vi "GUI_HPD_CCD.vi"() -> ()   [LabVIEW 2013]
uses:
  <vilib>/vision/Image Controls.llb/IMAQ Image.ctl
  Shared/GUI_Template/GUI_master/tcp new data cluster.ctl
  Shared/GUI_Template/GUI_master/tcp_new_data_event.ctl
panel:
  out "tcp data event":T1
  in  "Refresh Button":bool
  in  "Select device":string(combo)="FrogHPD"
  in  "stop":bool
  in  "trigger::1":bool caption="Trigger"
  in  "gain::1":dbl=0.001 caption="gain" min=12.0 max=400.0 format="%_4f"
  in  "centroidy::1":dbl=0.001 caption="centroid y" min=0.0 max=0.0 format="%_4f"
  in  "centroidx::1":dbl=0.001 caption="centroid x" min=0.0 max=0.0 format="%_4f"
  in  "exposure::1":dbl=0.001 caption="exposure" min=3.8e-05 max=1.0 format="%_4p"
  out "image::1":T2(plugin-control) caption="image"
  out "GUIdevice 1":string="HPD_CCD"
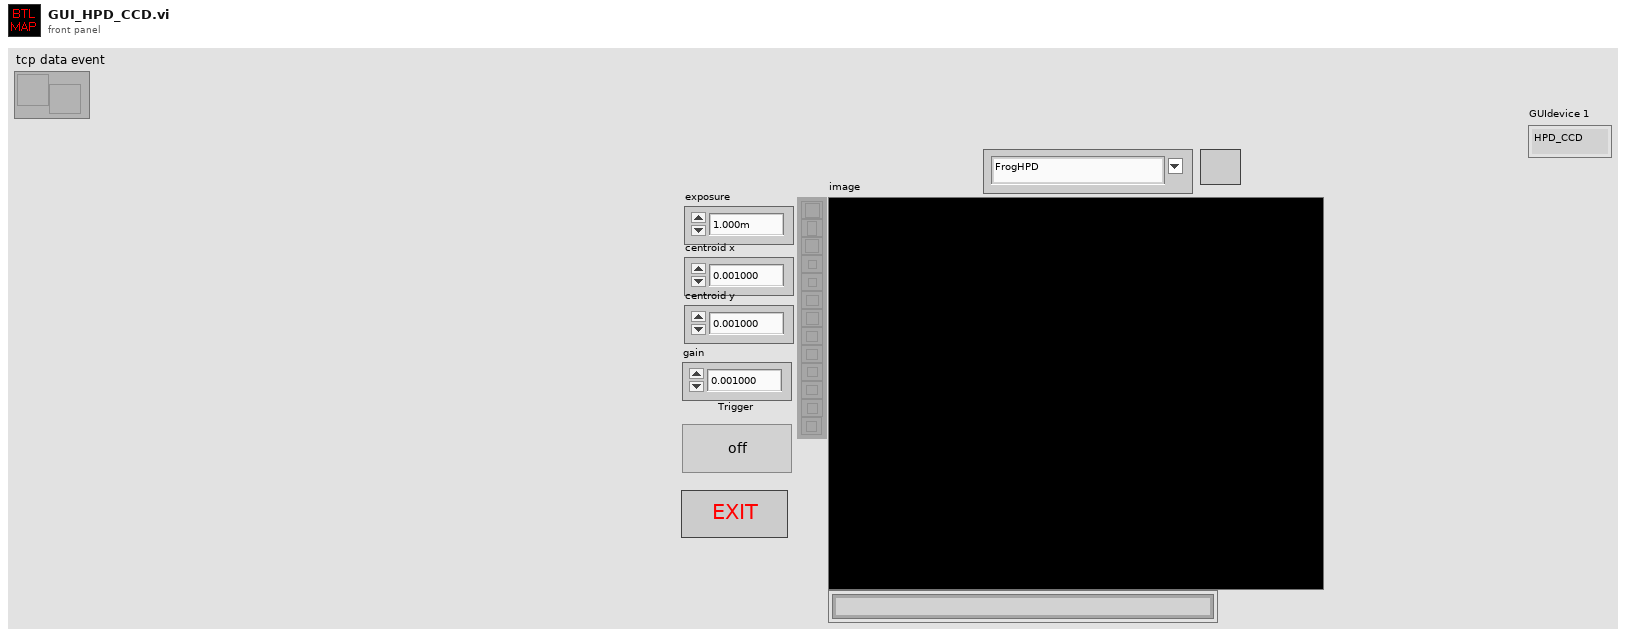
[diagram p1: front panel]
types:
  T1 = typedef "tcp_new_data_event.ctl" = refnum<user-event>
  T2 = typedef "IMAQ Image.ctl" = refnum<image>
  T3 = enum32{"invalid app kind", "Development System", "Run Time System", "Student Edition", "Embedded LabVIEW", "Evaluation", "Custom"}
  T4 = typedef "tcp new data cluster.ctl" = cluster{"EventEnum":enum16{"new data", "connection status update"}, "Device name":string}
  T5 = enum32{"Invalid", "Standard", "Closed", "Hidden", "Minimized", "Maximized"}
  T6 = cluster{"Core":cluster{"Current VI Reference":refnum<vi>, "Close Panel on Exit?":bool}, "Your Boolean data":bool, "Your string data":string, "SuperGUI":cluster{"STOP queue":refnum<queue>, "SuperGUI ref":refnum<vi>}}
  T7 = cluster{"STOP queue":refnum<queue>, "SuperGUI ref":refnum<vi>}
  T8 = cluster{"Current VI Reference":refnum<vi>, "Close Panel on Exit?":bool}
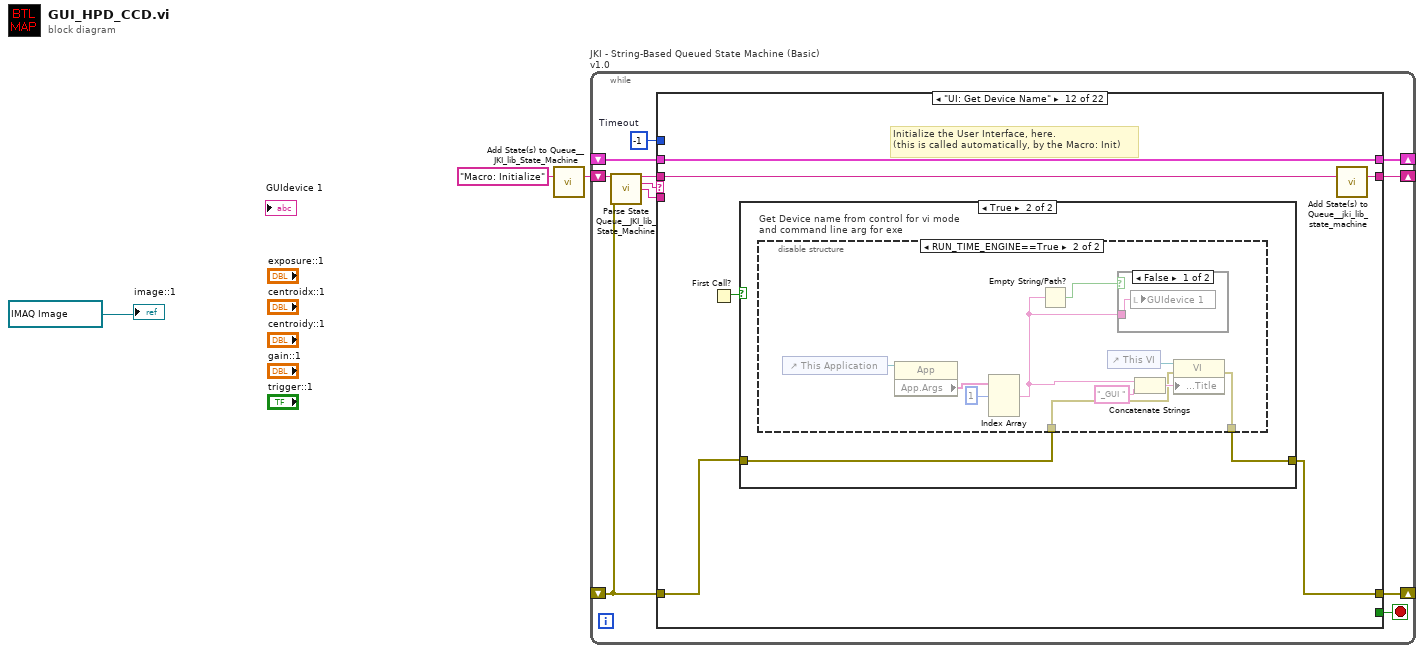
[diagram p0: block diagram]
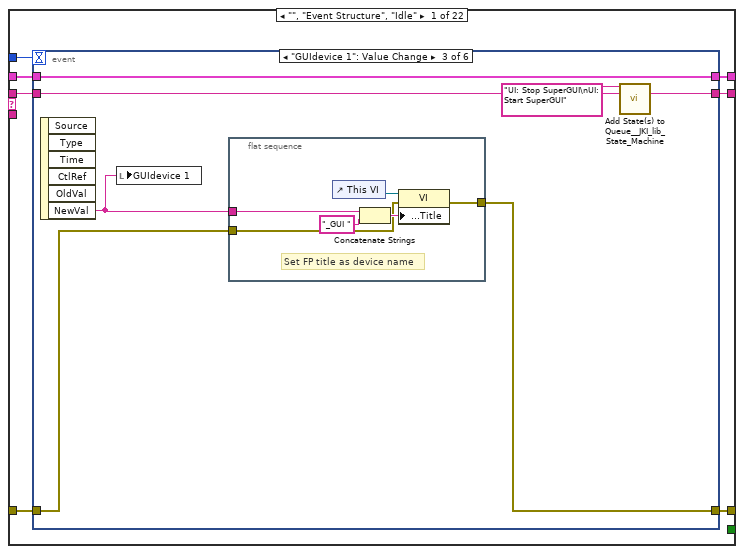
[diagram p2: hidden frame]
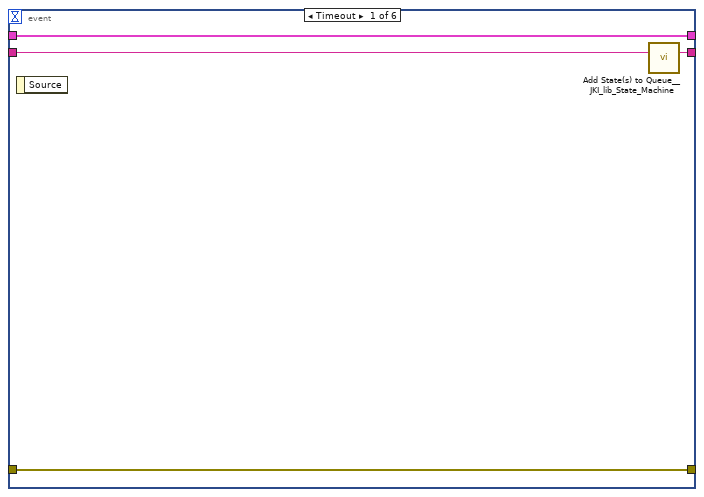
[diagram p3: hidden frame]
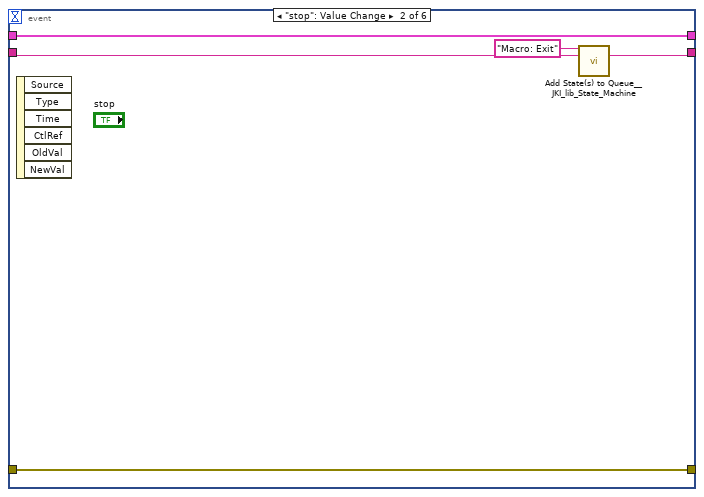
[diagram p4: hidden frame]
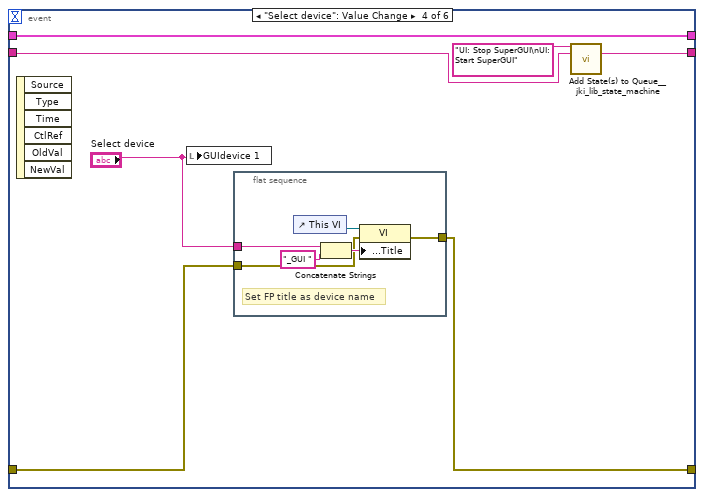
[diagram p5: hidden frame]
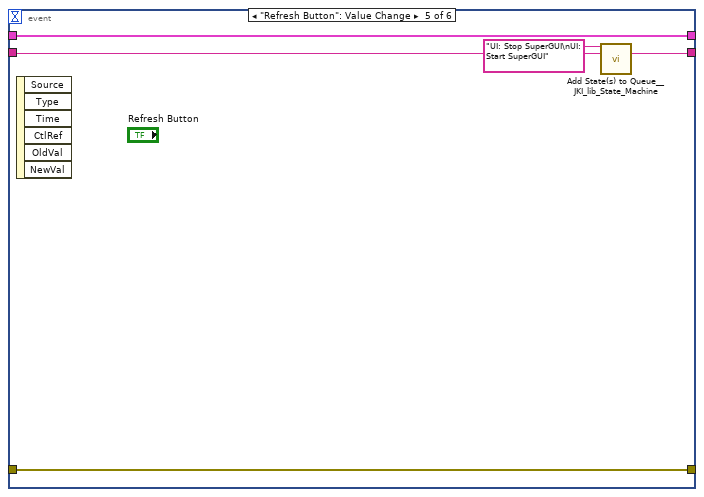
[diagram p6: hidden frame]
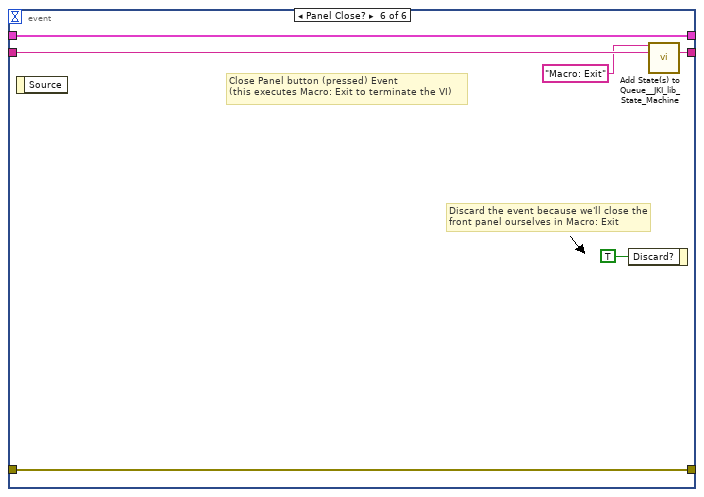
[diagram p7: hidden frame]
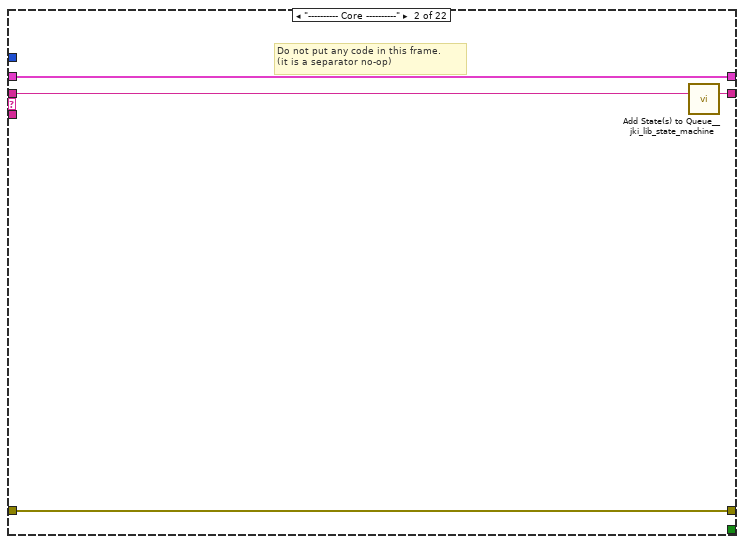
[diagram p8: hidden frame]
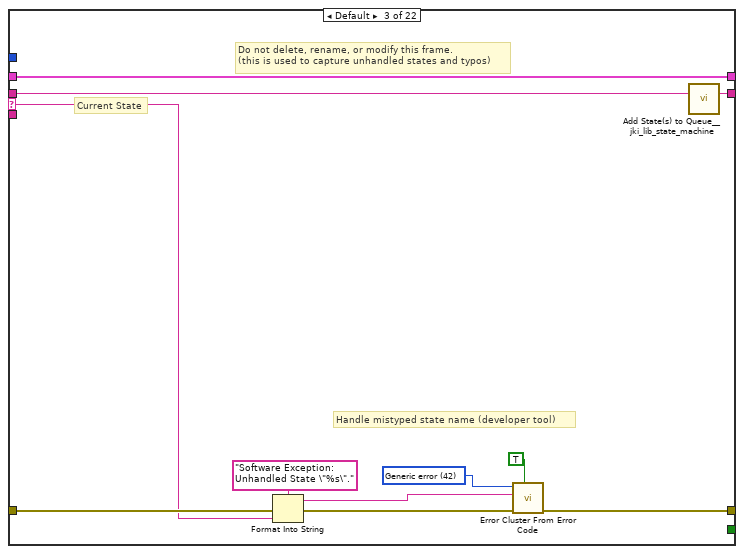
[diagram p9: hidden frame]
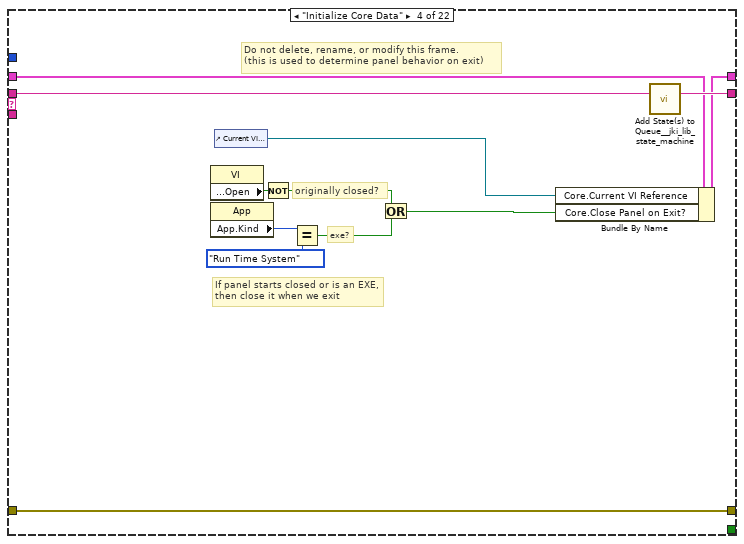
[diagram p10: hidden frame]
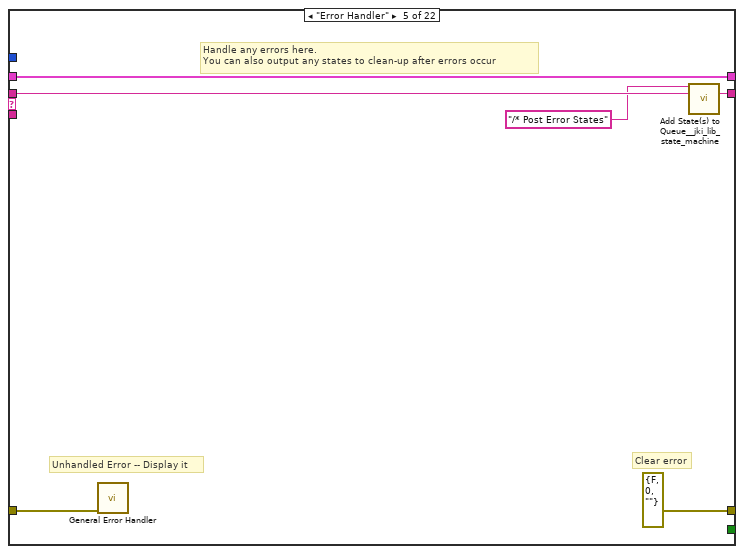
[diagram p11: hidden frame]
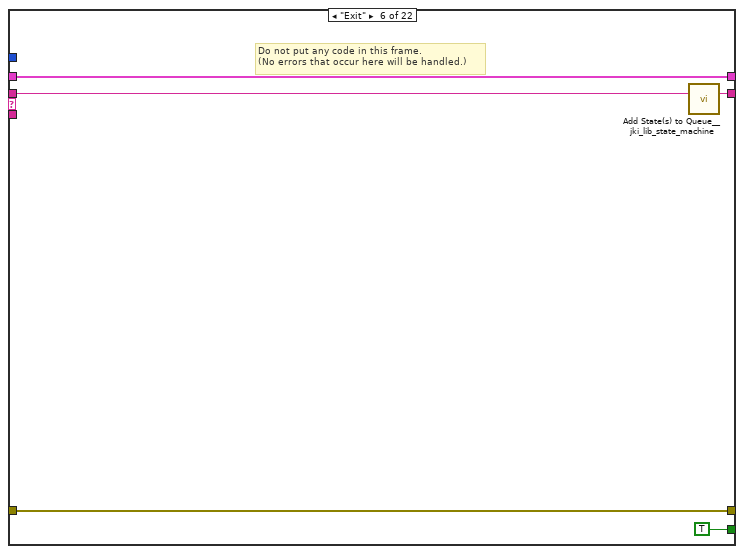
[diagram p12: hidden frame]
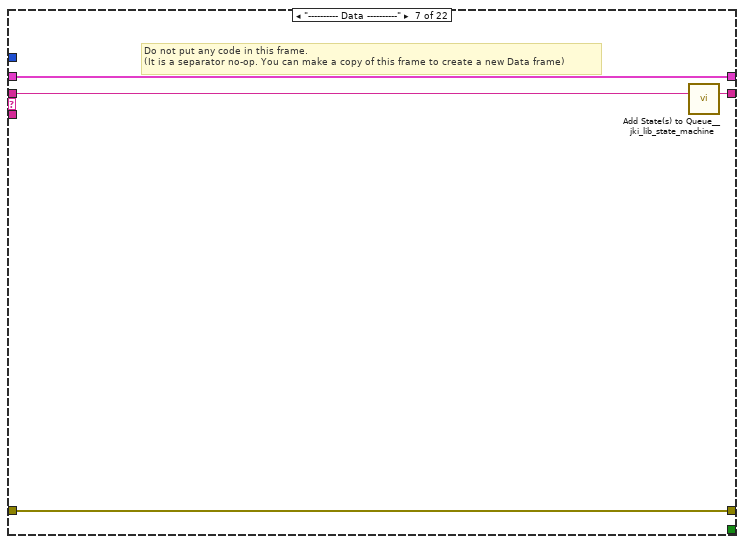
[diagram p13: hidden frame]
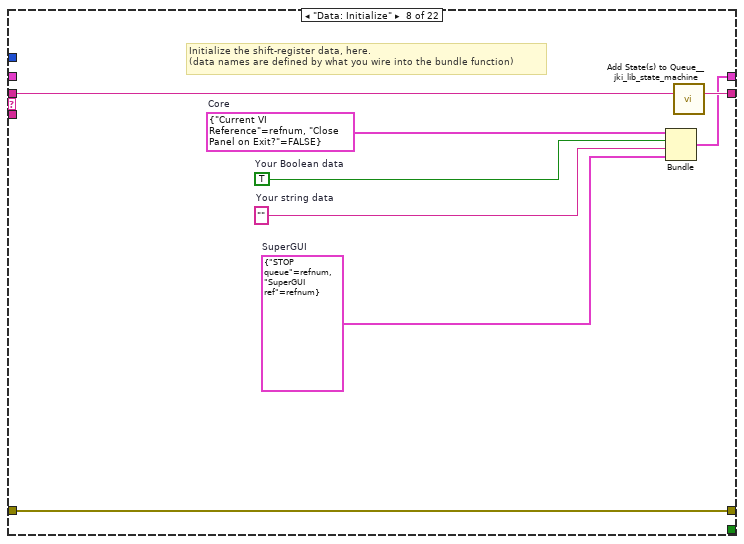
[diagram p14: hidden frame]
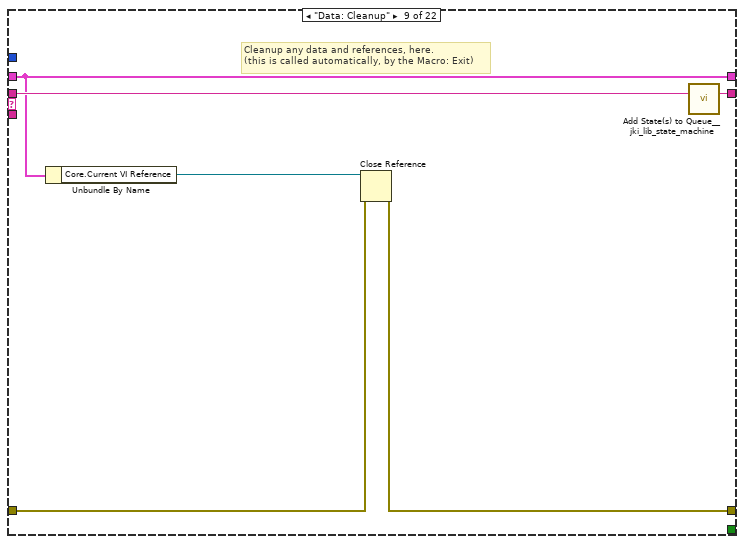
[diagram p15: hidden frame]
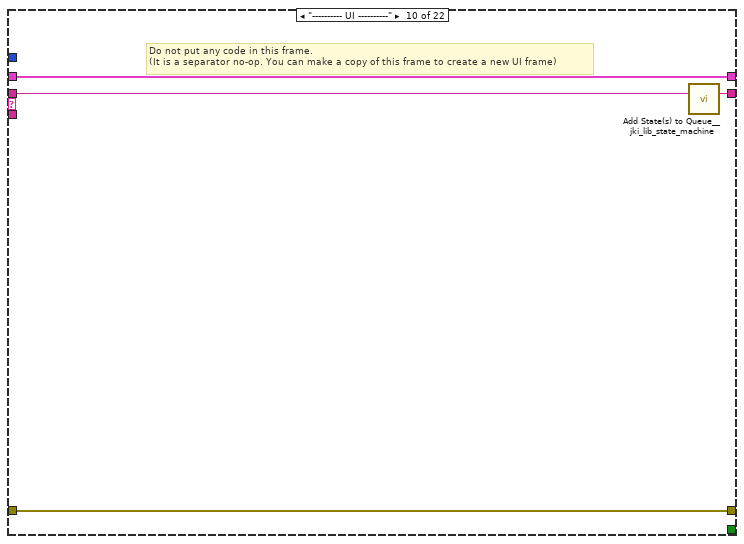
[diagram p16: hidden frame]
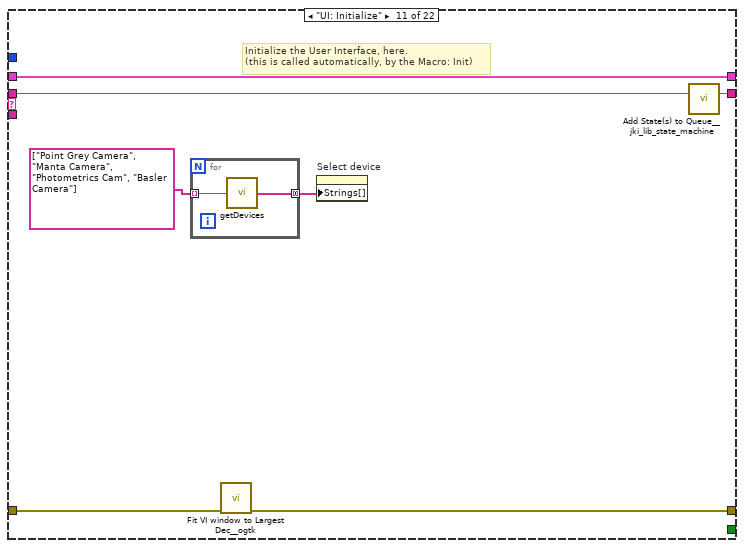
[diagram p17: hidden frame]
diagram:
  n1 = call <vilib>:"Add State(s) to Queue__JKI_lib_State_Machine.vi"("State(s) in (\"\")"="Macro: Initialize") -> ("States Out"=w2:string)  [unwired: 14 in]
  n2 = while "JKI - String-Based Queued State Machine (Basic) v1.0" {
    shift-right: [w7] -> _
    shift-left: _ -> [w6]
    shift-right: [w10] -> _
    shift-left: _ -> [w4]
    shift-right: [w9] -> _
    shift-left: w2 -> [w11]
    stop <- w8 stop-if-true
    w5 = -1  # Timeout
    n3 = call <vilib>:"Parse State Queue__JKI_lib_State_Machine.vi"("State Queue"=w11, "Error In (no error)"=w4) -> ("Remaining States"=w13:string, "Current State"=w14:string, "Arguments"=w12:string)  [unwired: 11 in]
    n4 = case shown="\"UI: Get Device Name\"" w14 {
      selector: w14 -> [_ _ w72 _ _ _ _ _ _ _ _ _ _ _ _ _ _ _ _ _ _ _]
      tunnel: w13 -> [w21 w71 w76 w94 w100 w105 w109 w117 w123 w127 w134 w142 w177 w185 w191 w202 w228 w233 w243 w247 w251 w255]
      tunnel: w12 -> [_ _ _ _ _ _ _ _ _ _ _ _ _ _ w186 w196 _ _ _ _ _ _]
      tunnel: w6 -> [w19 w68 w74 w85 w97 w103 w106 _ w118 w124 w132 w140 w168 w180 w189 w198 w225 w230 w240 w244 w248 w252]
      tunnel: [w18 w69 w78 w91 errorcluster {"status"=FALSE, "code"=0, "source"=""} ("error out") w102 w107 w114 w119 w125 w130 w137 w161 w178 w187 w199 w226 w231 w241 w245 w249 w253] -> w10
      tunnel: w4 -> [w17 w69 w77 w91 w96 w102 w107 w114 w120 w125 w131 w138 w162 w179 w188 w200 w226 w231 w241 w245 w249 w253]
      tunnel: [w20 w70 w75 w93 w99 w104 w108 w116 w122 w126 w133 w141 w176 w184 w190 w201 w227 w232 w242 w246 w250 w254] -> w9
      tunnel: [_ _ _ _ _ TRUE _ _ _ _ _ _ _ _ _ _ _ _ _ _ _ _] -> w8
      tunnel: [w16 w68 w74 w92 w97 w103 w106 w115 w118 w124 w132 w140 w167 w180 w189 w198 w225 w230 w240 w244 w248 w252] -> w7
      tunnel: w5 -> [w15 _ _ _ _ _ _ _ _ _ _ _ _ _ _ _ _ _ _ _ _ _]
      frame "", "Event Structure", "Idle" {
        n5 = event shown="[2] \"GUIdevice 1\": Value Change" {
          selector: _ -> [_ _ _ _ _ _]
          dyn-events: _ -> [_ _ _ _ _ _]
          timeout: w15 -> [_ _ _ _ _ _]
          tunnel: w21 -> [w25 w28 w34 w46 w59 w67]
          tunnel: [w24 w27 w33 w45 w58 w66] -> w20
          tunnel: w19 -> [w22 w30 w37 w50 w61 w64]
          tunnel: [w23 w29 w35 w48 w60 w65] -> w18
          tunnel: w17 -> [w23 w29 w36 w49 w60 w65]
          tunnel: [w22 w30 w37 w50 w61 w64] -> w16
          event Timeout {
            n6 = event-data() -> ()  [unwired: 1 in, 1 out]
            n7 = call <vilib>:"Add State(s) to Queue__JKI_lib_State_Machine.vi"("State(s) in (\"\")"=w25) -> ("States Out"=w24:string)  [unwired: 14 in]
          }
          event "stop": Value Change {
            n8 = event-data() -> ()  [unwired: 1 in, 6 out]
            n9 = call <vilib>:"Add State(s) to Queue__JKI_lib_State_Machine.vi"("State(s) in Front (\"\")"="Macro: Exit", "State(s) in (\"\")"=w28) -> ("States Out"=w27:string)  [unwired: 13 in]
          }
          event "GUIdevice 1": Value Change {
            n10 = event-data() -> ("NewVal"=w31:string)  [unwired: 1 in, 5 out]
            n11 = local write "GUIdevice 1"(w31) -> ()
            n12 = flat-sequence {
              tunnel: [w40] -> w35
              tunnel: w36 -> [w39]
              tunnel: w31 -> [w38]
              frame #0 {
                # "Set FP title as device name"
                n13 = control-ref of="This VI"() -> (w43:refnum<vi>)
                n14 = Concatenate Strings(w38, "_GUI ") -> (w42:string)
                n15 = property class="VI"(reference=w43, error in=w39, "Front Panel.Title"=w42) -> (error out=w40:errorcluster)  [unwired: 1 out]
              }
            }
            n16 = call <vilib>:"Add State(s) to Queue__JKI_lib_State_Machine.vi"("State(s) in Front (\"\")"="UI: Stop SuperGUI\nUI: Start SuperGUI", "State(s) in (\"\")"=w34) -> ("States Out"=w33:string)  [unwired: 13 in]
          }
          event "Select device": Value Change {
            n17 = event-data() -> ()  [unwired: 1 in, 6 out]
            n18 = local write "GUIdevice 1"("Select device") -> ()
            n19 = flat-sequence {
              tunnel: [w53] -> w48
              tunnel: w49 -> [w52]
              tunnel: "Select device" -> [w51]
              frame #0 {
                # "Set FP title as device name"
                n20 = control-ref of="This VI"() -> (w56:refnum<vi>)
                n21 = Concatenate Strings(w51, "_GUI ") -> (w55:string)
                n22 = property class="VI"(reference=w56, error in=w52, "Front Panel.Title"=w55) -> (error out=w53:errorcluster)  [unwired: 1 out]
              }
            }
            n23 = call <vilib>:"Add State(s) to Queue__jki_lib_state_machine.vi"("State(s) in Front (\"\")"="UI: Stop SuperGUI\nUI: Start SuperGUI", "State(s) in (\"\")"=w46) -> ("States Out"=w45:string)  [unwired: 13 in]
          }
          event "Refresh Button": Value Change {
            n24 = event-data() -> ()  [unwired: 1 in, 6 out]
            n25 = call <vilib>:"Add State(s) to Queue__JKI_lib_State_Machine.vi"("State(s) in Front (\"\")"="UI: Stop SuperGUI\nUI: Start SuperGUI", "State(s) in (\"\")"=w59) -> ("States Out"=w58:string)  [unwired: 13 in]
          }
          event Panel Close? {
            # "Discard the event because we'll close the front panel ourselves in Macro: Exit"
            # "Close Panel button (pressed) Event\n(this executes Macro: Exit to terminate the VI)"
            n26 = event-data() -> ()  [unwired: 1 in, 1 out]
            n27 = event-data("Discard?"=TRUE) -> ()  [unwired: 1 in, 1 out]
            n28 = call <vilib>:"Add State(s) to Queue__JKI_lib_State_Machine.vi"("State(s) in Front (\"\")"="Macro: Exit", "State(s) in (\"\")"=w67) -> ("States Out"=w66:string)  [unwired: 13 in]
          }
        }
      }
      frame "---------- Core ----------" {
        # "Do not put any code in this frame.\n(it is a separator no-op)"
        n29 = call <vilib>:"Add State(s) to Queue__jki_lib_state_machine.vi"("State(s) in (\"\")"=w71) -> ("States Out"=w70:string)  [unwired: 14 in]
      }
      frame Default {
        w81 = 42 items=["No error", "Argument error", "Memory is full", "Out of zone", "End of file", "File already open", "Generic file I/O error", "File not found", "File permission error", "Disk is full", "Duplicate path", "Too many files open", "System feature not enabled", "Resource file not found", "Cannot add resource", "Resource not found", "Image not found", "Image memory error", "Pen does not exist", "Config type invalid", "Config token not found", "Config parse error", "Config memory error", "Bad external code format", "Bad external code offset", "External code not present", "Null window", "Destroy window error", "Null menu", "Print aborted", "Bad print record", "Print driver error", "Windows error during printing", "Memory error during printing", "Print dialog error", "Generic print error", "Invalid device refnum", "Device not found", "Device parameter error", "Device unit error", "Cannot open device", "Device call aborted", "Generic error", "Cancelled by user", "Object ID too low", "Object ID too high", "Object not in heap", "Unknown heap", "Unknown object (invalid DefProc)", "Unknown object (DefProc not in table)", "Message out of range", "Invalid (null) method", "Unknown message", "Manager call not supported", "Bad address", "Network operation in progress", "Network operation timed out", "Connection is busy", "Network attribute not supported", "Network error", "Address in use", "System out of memory", "Connection aborted", "Connection refused", "Not connected", "Already connected", "Connection closed", "Initialization error (interapplication manager)", "Bad occurrence", "Wait on unbound occurrence handler", "Occurrence queue overflow", "Datalog type conflict", "Unused", "Unrecognized type (interapplication manager)", "Memory corrupt", "Failed to make temporary DLL", "Old CIN version", "Drag socket not found", "Failed to load drop-object", "Failed to register OLE object", "Failed to release OLE object", "Format specifier type mismatch", "Unknown format specifier", "Too few format specifiers", "Too many format specifiers", "Scan failed", "Newer CIN version", "Error converting to variant", "Runtime menu error", "Password tampered", "Variant attribute not found", "Incompatible variant data type", "Event data is not available", "Event Store is not present", "Occurrence is not found", "Event Queue is not created", "Event info is not available", "Refnum passed is NULL", "Error retrieving Class GUID", "Error retrieving CoClass GUID", "Error retrieving TypeLib GUID.", "Bad built application magic bytes.", "Specific driver is different from the specific driver associated with the Logical Name.", "There is no session opened to the class driver.", "Max Error", "MAX - Error with config objects", "MAX - Error loading configuration", "MAX - Group not supported"]
        # "Current State"
        # "Do not delete, rename, or modify this frame.\n(this is used to capture unhandled states and typos)"
        # "Handle mistyped state name (developer tool)"
        n30 = Format Into String(format string="Software Exception: Unhandled State \"%s\"." ("message"), error in=w77, w72) -> (resulting string=w80:string, error out=w79:errorcluster)  [unwired: 1 in]
        n31 = call <vilib>:"Error Cluster From Error Code.vi"("show call chain? (False)"=TRUE, "error in (no error)"=w79, "error message (\"\")"=w80, "error code (0)"=w81) -> ("error out"=w78:errorcluster)  [unwired: 5 in]
        n32 = call <vilib>:"Add State(s) to Queue__jki_lib_state_machine.vi"("State(s) in (\"\")"=w76) -> ("States Out"=w75:string)  [unwired: 14 in]
      }
      frame "Initialize Core Data" {
        # "Do not delete, rename, or modify this frame.\n(this is used to determine panel behavior on exit)"
        # "originally closed?"
        # "exe?"
        # "If panel starts closed or is an EXE, then close it when we exit"
        n33 = property class="VI"() -> ("Front Panel.Open"=w90:bool)  [unwired: 2 in, 2 out]
        n34 = property class="App"() -> ("App.Kind"=w89:T3)  [unwired: 2 in, 2 out]
        n35 = control-ref of="Current VI Reference"() -> (w83:refnum<vi>)
        n36 = Not(x=w90) -> (.not. x?=w87:bool)
        n37 = Equal?(x=w89, y=T3."Run Time System" ("Application:Kind")) -> (x = y?=w86:bool)
        n38 = Or(x=w87, y=w86) -> (x .or. y?=w84:bool)
        n39 = Bundle By Name(cluster=w85, "Core.Current VI Reference"=w83, "Core.Close Panel on Exit?"=w84) -> (w92:T6)
        n40 = call <vilib>:"Add State(s) to Queue__jki_lib_state_machine.vi"("State(s) in (\"\")"=w94) -> ("States Out"=w93:string)  [unwired: 14 in]
      }
      frame "Error Handler" {
        # "Unhandled Error -- Display it"
        # "Handle any errors here.\nYou can also output any states to clean-up after errors occur"
        # "Clear error"
        n41 = call <vilib>:"General Error Handler.vi"("error in (no error)"=w96) -> ()  [unwired: 10 in, 5 out]
        n42 = call <vilib>:"Add State(s) to Queue__jki_lib_state_machine.vi"("State(s) in Front (\"\")"="/* Post Error States", "State(s) in (\"\")"=w100) -> ("States Out"=w99:string)  [unwired: 13 in]
      }
      frame "Exit" {
        # "Do not put any code in this frame.\n(No errors that occur here will be handled.)"
        n43 = call <vilib>:"Add State(s) to Queue__jki_lib_state_machine.vi"("State(s) in (\"\")"=w105) -> ("States Out"=w104:string)  [unwired: 14 in]
      }
      frame "---------- Data ----------" {
        # "Do not put any code in this frame.\n(It is a separator no-op. You can make a copy of this frame to create a new Data frame)"
        n44 = call <vilib>:"Add State(s) to Queue__jki_lib_state_machine.vi"("State(s) in (\"\")"=w109) -> ("States Out"=w108:string)  [unwired: 14 in]
      }
      frame "Data: Initialize" {
        w110 = T7 {"STOP queue"=refnum, "SuperGUI ref"=refnum}  # SuperGUI
        w111 = T8 {"Current VI Reference"=refnum, "Close Panel on Exit?"=FALSE}  # Core
        w113 = TRUE  # Your Boolean data
        w112 = ""  # Your string data
        # "Initialize the shift-register data, here.\n(data names are defined by what you wire into the bundle function)"
        n45 = Bundle("Core"=w111, "Your Boolean data"=w113, "Your string data"=w112, "SuperGUI"=w110) -> (w115:T6)  [unwired: 1 in]
        n46 = call <vilib>:"Add State(s) to Queue__jki_lib_state_machine.vi"("State(s) in (\"\")"=w117) -> ("States Out"=w116:string)  [unwired: 14 in]
      }
      frame "Data: Cleanup" {
        # "Cleanup any data and references, here.\n(this is called automatically, by the Macro: Exit)"
        n47 = Unbundle By Name(w118) -> ("Core.Current VI Reference"=w121:refnum<vi>)
        n48 = Close Reference(reference=w121, error in (no error)=w120) -> (error out=w119:errorcluster)
        n49 = call <vilib>:"Add State(s) to Queue__jki_lib_state_machine.vi"("State(s) in (\"\")"=w123) -> ("States Out"=w122:string)  [unwired: 14 in]
      }
      frame "---------- UI ----------" {
        # "Do not put any code in this frame.\n(It is a separator no-op. You can make a copy of this frame to create a new UI frame)"
        n50 = call <vilib>:"Add State(s) to Queue__jki_lib_state_machine.vi"("State(s) in (\"\")"=w127) -> ("States Out"=w126:string)  [unwired: 14 in]
      }
      frame "UI: Initialize" {
        # "Initialize the User Interface, here.\n(this is called automatically, by the Macro: Init)"
        n51 = for {
          tunnel: string[] ["Point Grey Camera", "Manta Camera", "Photometrics Cam", "Basler Camera"] -> [w136] mode=indexing
          tunnel: [w135] -> w128 mode=concatenating
          n52 = call "getDevices.vi"("Device Class"=w136) -> ("All Devices"=w135:string[])
        }
        n53 = call <userlib>:"Fit VI window to Largest Dec__ogtk.vi"("error in (no error)"=w131) -> ("error out"=w130:errorcluster)  [unwired: 5 in, 1 out]
        n54 = property on="Select device" class="CmbBox"("Strings[]"=w128) -> ()  [unwired: 2 in, 2 out]
        n55 = call <vilib>:"Add State(s) to Queue__jki_lib_state_machine.vi"("State(s) in (\"\")"=w134) -> ("States Out"=w133:string)  [unwired: 14 in]
      }
      frame "UI: Get Device Name" {
        # "Initialize the User Interface, here.\n(this is called automatically, by the Macro: Init)"
        n56 = First Call?() -> (First Call?: T/F=w139:bool)
        n57 = case shown="True" w139 {
          tunnel: w138 -> [w143 w145]
          tunnel: [w143 w144] -> w137
          frame False {
          }
          frame True {
            n58 = disable-structure "Get Device name from control for vi mode\nand command line arg for exe" shown="RUN_TIME_ENGINE==True" {
              disable-tunnel: w145 -> [w146 w148]
              disable-tunnel: [w146 w147] -> w144
              frame condition #0 (active) {
              }
              frame condition #1 {
                n59 = control-ref of="This Application"() -> (w156:refnum<vi>)
                n60 = property class="App"(reference=w156) -> ("App.Args"=w155:string[])  [unwired: 1 in, 2 out]
                n61 = Index Array(array=w155, index #1=1 ("index")) -> (element #1=w149:string)  [unwired: 2 in, 2 out]
                n62 = Empty String/Path?(string/path=w149) -> (empty?=w153:bool)
                n63 = control-ref of="This VI"() -> (w152:refnum<vi>)
                n64 = case shown="False" w153 {
                  tunnel: w149 -> [w157 _]
                  frame False {
                    n65 = local write "GUIdevice 1"(w157) -> ()
                  }
                  frame True {
                  }
                }
                n66 = Concatenate Strings(w149, "_GUI ") -> (w151:string)
                n67 = property class="VI"(reference=w152, error in=w148, "Front Panel.Title"=w151) -> (error out=w147:errorcluster)  [unwired: 1 out]
              }
            }
          }
        }
        n68 = call <vilib>:"Add State(s) to Queue__jki_lib_state_machine.vi"("State(s) in (\"\")"=w142) -> ("States Out"=w141:string)  [unwired: 14 in]
      }
      frame "UI: Start SuperGUI" {
        # "create stop queue for supergui and its clones"
        # "x100 abort will be dependent on caller VI\nx80 abort will be independent of caller vi, this will abort vi when labview is closed."
        # "Start SuperGUI asynchronous way"
        n69 = vi-ref "GUI_Master_subvi_reentrant_queues.vi"() -> (w160:refnum<vi>)
        n70 = property class="VI"(reference=w160) -> ("Path"=w159:path)  [unwired: 1 in, 2 out]
        n71 = Create User Event(user event datatype=T4 {"EventEnum"=enum."new data", "Device name"="Device name"} ("New Event"), error in=w162) -> (user event=w163:refnum<user-event>, error out=w169:errorcluster)
        "tcp data event" <- w163
        n72 = control-ref of="This Application"() -> (w166:refnum<vi>)
        n73 = control-ref of="This VI"() -> (w165:refnum<vi>)
        n74 = Open VI Reference(type specifier VI Refnum (for type only)=refnum<vi> refnum, vi path=w159, options=256) -> (vi reference=w175:refnum<vi>, error out=w174:errorcluster)  [unwired: 3 in]
        n75 = register-events(w163) -> ()  [unwired: 2 in, 2 out]
        n76 = call "supergui create stop queue.vi"() -> ("STOP Queue out"=w171:refnum<queue>)  [unwired: 11 in]
        n77 = Current VI's Menubar() -> (w164:refnum<k9>)
        n78 = call-by-ref "Start Asynchronous Call"(reference=w175, error in=w174, "STOP Queue in"=w171, "This Application"=w166, 8:"error in (no error)"=w169, "tcp data event"=w163, "Caller menu reference"=w164, "Caller VI ref"=w165) -> (reference out=w158:refnum<vi>, error out=w161:errorcluster)  [unwired: 5 in, 1 out]
        n79 = Bundle By Name(cluster=w168, "SuperGUI.SuperGUI ref"=w158, "SuperGUI.STOP queue"=w171) -> (w167:T6)
        n80 = call <vilib>:"Add State(s) to Queue__jki_lib_state_machine.vi"("State(s) in (\"\")"=w177) -> ("States Out"=w176:string)  [unwired: 14 in]
      }
      frame "UI: Stop SuperGUI" {
        # "Stop Supergui Clone and wait until it exit properly"
        n81 = Unbundle By Name(w180) -> ("SuperGUI.SuperGUI ref"=w182:refnum<vi>, "SuperGUI.STOP queue"=w181:refnum<queue>)
        n82 = Release Queue(queue=w181, error in (no error)=w179) -> (error out=w183:errorcluster)  [unwired: 1 in, 2 out]
        n83 = call-by-ref "Wait On Asynchronous Call"(reference=w182, error in=w183) -> ("error out"=w178:errorcluster)  [unwired: 11 in, 2 out]
        n84 = call <vilib>:"Add State(s) to Queue__jki_lib_state_machine.vi"("State(s) in (\"\")"=w185) -> ("States Out"=w184:string)  [unwired: 14 in]
      }
      frame "UI: Cursor Set" {
        # "Argument"
        # "Set and Unset Cursor Busy.\n(Usage: \"UI: Cursor Set >> Busy|Idle\")"
        n85 = case shown="\"Idle\", Default" w186 {
          tunnel: w188 -> [w193 w195]
          tunnel: [w192 w194] -> w187
          frame "Idle", Default {
            n86 = call <vilib>:"Unset Busy.vi"("error in (no error)"=w193) -> ("error out"=w192:errorcluster)  [unwired: 10 in]
          }
          frame "Busy" {
            n87 = call <vilib>:"Set Busy.vi"("error in (no error)"=w195) -> ("error out"=w194:errorcluster)  [unwired: 9 in, 1 out]
          }
        }
        n88 = call <vilib>:"Add State(s) to Queue__jki_lib_state_machine.vi"("State(s) in (\"\")"=w191) -> ("States Out"=w190:string)  [unwired: 14 in]
      }
      frame "UI: Front Panel State" {
        # "Argument"
        # "Set Front Panel Open or Closed\n(Usage: \"UI: Front Panel State >> Open|Close\")"
        n89 = Unbundle By Name(w198) -> ("Core.Current VI Reference"=w197:refnum<vi>)
        n90 = case shown="\"Open\", Default" w196 {
          tunnel: w200 -> [w206 w219]
          tunnel: [w208 w220] -> w199
          tunnel: w197 -> [w207 w217]
          frame "Open", Default {
            n91 = property class="VI"(reference=w207, error in=w206) -> (reference out=w204:refnum<vi>, error out=w205:errorcluster, "Front Panel.Open"=w203:bool)
            n92 = case shown="False" w203 {
              tunnel: [w211 w214] -> w208
              tunnel: w205 -> [w210 w214]
              tunnel: w204 -> [w209 _]
              frame False {
                n93 = invoke class="VI" method="FP.Open"(reference=w209, error in=w210, "Activate"=TRUE, "State"=T5."Standard") -> (error out=w211:errorcluster)  [unwired: 1 in, 4 out]
              }
              frame True {
              }
            }
          }
          frame "Close" {
            n94 = property class="VI"(reference=w217, error in=w219) -> (reference out=w216:refnum<vi>, error out=w218:errorcluster, "Front Panel.Open"=w215:bool)
            n95 = case shown="True" w215 {
              tunnel: [w221 w224] -> w220
              tunnel: w218 -> [w221 w223]
              tunnel: w216 -> [_ w222]
              frame False {
              }
              frame True {
                n96 = invoke class="VI" method="FP.Close"(reference=w222, error in=w223) -> (error out=w224:errorcluster)  [unwired: 1 in, 2 out]
              }
            }
          }
        }
        n97 = call <vilib>:"Add State(s) to Queue__jki_lib_state_machine.vi"("State(s) in (\"\")"=w202) -> ("States Out"=w201:string)  [unwired: 14 in]
      }
      frame "---------- Macro ----------" {
        # "Do not put any code in this frame.\n(It is a separator no-op. You can make a copy of this frame to create a new Macro frame)"
        n98 = call <vilib>:"Add State(s) to Queue__jki_lib_state_machine.vi"("State(s) in (\"\")"=w228) -> ("States Out"=w227:string)  [unwired: 14 in]
      }
      frame "Macro: Initialize" {
        # "Initialization Macro\n(This is called once, when the VI starts)"
        n99 = call <vilib>:"Add State(s) to Queue__jki_lib_state_machine.vi"("State(s) in Front (\"\")"="Data: Initialize\nInitialize Core Data\nUI: Initialize\nUI: Get Device Name\nUI: Start SuperGUI\nUI: Front Panel State >> Open", "State(s) in (\"\")"=w233) -> ("States Out"=w232:string)  [unwired: 13 in]
      }
      frame "Macro: Exit" {
        # "Exit Macro\n(This is called once, when the VI exits)"
        n100 = Unbundle By Name(w240) -> ("Core.Close Panel on Exit?"=w239:bool)
        n101 = Select(t="UI: Front Panel State >> Close", s=w239, f="") -> (s? t:f=w236:string)
        n102 = call <vilib>:"Add State(s) to Queue__jki_lib_state_machine.vi"("State(s) in (\"\")"=w236, "State(s) at Back (\"\")"="Data: Cleanup\nExit") -> ("States Out"=w234:string)  [unwired: 13 in]
        n103 = call <vilib>:"Add State(s) to Queue__jki_lib_state_machine.vi"("State(s) in Front (\"\")"=w234, "State(s) in (\"\")"=w243) -> ("States Out"=w242:string)  [unwired: 13 in]
      }
      frame "---------- New Category ----------" {
        # "Template Separator\n(You can make a copy of, or modify, this frame)"
        n104 = call <vilib>:"Add State(s) to Queue__jki_lib_state_machine.vi"("State(s) in (\"\")"=w247) -> ("States Out"=w246:string)  [unwired: 14 in]
      }
      frame "New Category: 1" {
        # "Your code here.\n(You can make a copy of, or modify, this frame)"
        n105 = call <vilib>:"Add State(s) to Queue__jki_lib_state_machine.vi"("State(s) in (\"\")"=w251) -> ("States Out"=w250:string)  [unwired: 14 in]
      }
      frame "New Category: 2" {
        # "Your code here.\n(You can make a copy of, or modify, this frame)"
        n106 = call <vilib>:"Add State(s) to Queue__jki_lib_state_machine.vi"("State(s) in (\"\")"=w255) -> ("States Out"=w254:string)  [unwired: 14 in]
      }
    }
  }
  "image::1" <- T2 refnum ("image::1")
